vi "Acquisition-Exit.vi"(8 "error in (no error)":errorcluster, 9 "FPGA Ref":T6, 10 "Logging queue element in":T1 {"Ref Dwell time (us)" format="%#.6g"; "Frame Size" items=["100X100"=100, "128X128"=128, "200X200"=200, "256X256"=256, "512X512"=512, "1024x1024"=1024, "2048x2048"=2048]; "Dwell time (us)" format="%#.6g"}, 11 "Logging queue in":T5) -> (0 "error out":errorcluster, 2 "Logging queue element":T1={"Imaging Protocol"=enum."Live Imaging", "Number of Trials"=0, "Frame Size"=512, "# Averaged frames"=0, "Dwell time (us)"=0.0, "Index of Z-plane"=0, "Timelapse?"=FALSE, "Logging process is active"=FALSE, "Speed logging enabled"=FALSE, "tdms file ref"=refnum, "path"=path "", "Trial Number"=0, "Expected # points acquired"=FALSE, "Manually stopped"=FALSE, "Last trial"=FALSE, "Ch0 data"=[], "Ch1 data"=[], "Ref Data"=[], "Ref Frame Time"=[], "Image Time"=[], "Continuous Time"=[], "Ref X Length"=0, "Ref Y Length"=0, "# Ref Averaged frames"=0, "Ref Dwell time (us)"=0.0, "Points acquired"={"Ch0 last trial"=0, "Ch1 last trial"=0, "All trials"=0}, "HW Timings File"=refnum} {"Ref Dwell time (us)" format="%#.6g"; "Frame Size" items=["100X100"=100, "128X128"=128, "200X200"=200, "256X256"=256, "512X512"=512, "1024x1024"=1024, "2048x2048"=2048]; "Dwell time (us)" format="%#.6g"}, 3 "Logging queue out":T5)   [LabVIEW 2017]
doc: "Executes the required code on acquisition exit.\nThis may be at the end of live imaging or at the end of each functional acquisition trial."
uses:
  RIG-SPECIFIC FILES/FPGA Refs/FPGA Ref.ctl
  Typedefs/Logging queue element.ctl
  Typedefs/Imaging Protocols enum.ctl
  Typedefs/Frame Size.ctl
  Typedefs/Acquired points count.ctl
  Typedefs/Data queue ref.ctl
panel:
  in  "Debugging delay":u32
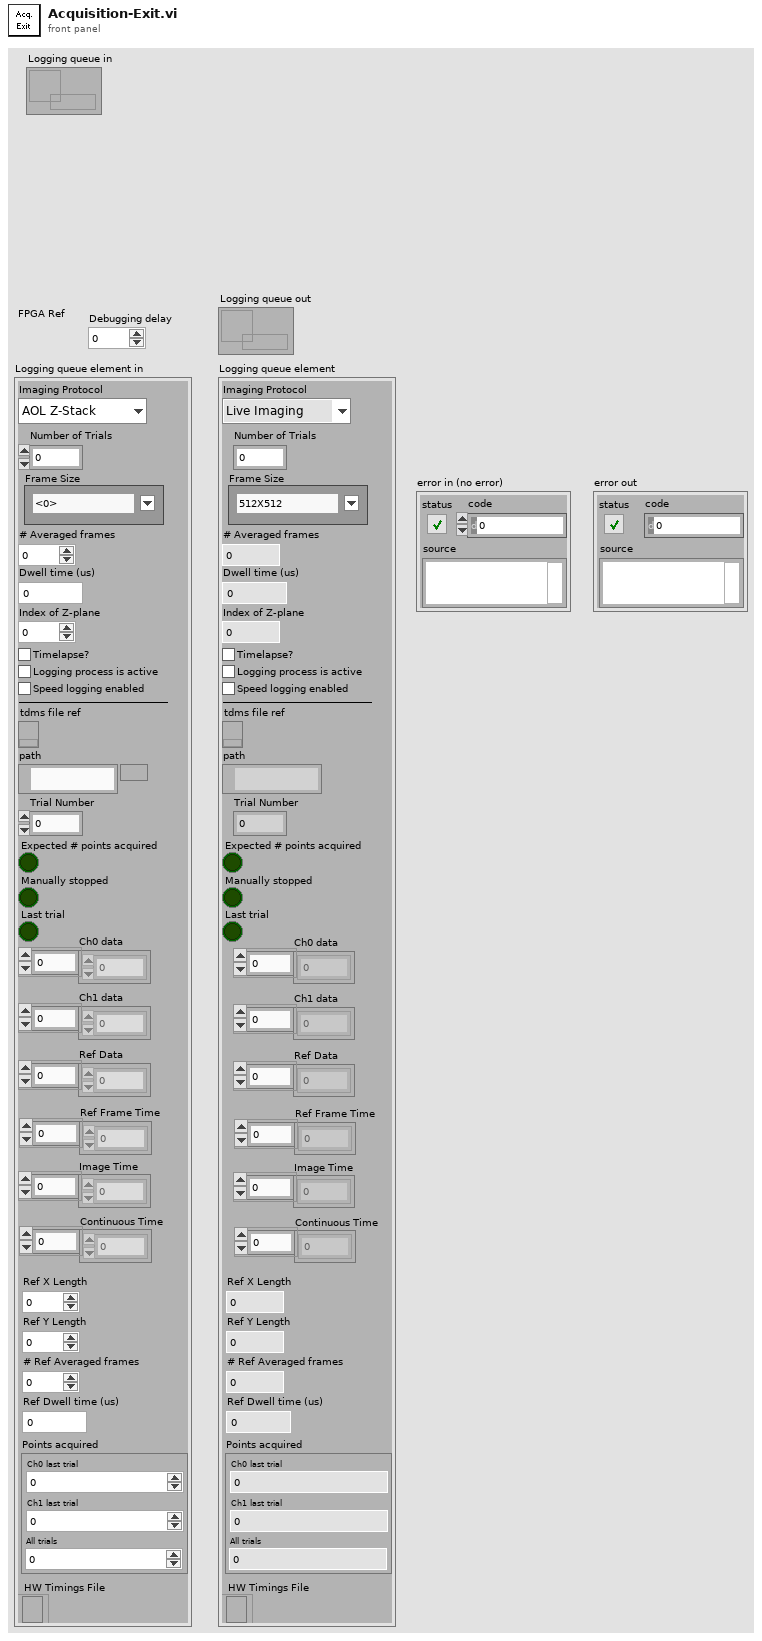
[diagram p1: front panel]
types:
  T1 = typedef "Logging queue element.ctl" = cluster{"Imaging Protocol":T2, "Number of Trials":u16, "Frame Size":T3, "# Averaged frames":u16, "Dwell time (us)":dbl, "Index of Z-plane":i32, "Timelapse?":bool, "Logging process is active":bool, "Speed logging enabled":bool, "tdms file ref":refnum<k34>, "path":path, "Trial Number":i32, "Expected # points acquired":bool, "Manually stopped":bool, "Last trial":bool, "Ch0 data":u32[], "Ch1 data":u32[], "Ref Data":u32[], "Ref Frame Time":u64[], "Image Time":u64[], "Continuous Time":u64[], "Ref X Length":u16, "Ref Y Length":u16, "# Ref Averaged frames":u16, "Ref Dwell time (us)":dbl, "Points acquired":T4, "HW Timings File":refnum<file>}
  T2 = typedef "Imaging Protocols enum.ctl" = enum16{"AOL Z-Stack", "Motor Z Stack", "Functional Acquisition", "Single Plane Acquisition", "Volume Acquisition", "Live Imaging", "Live Plane Imaging", "Live Volume Imaging"}
  T3 = typedef "Frame Size.ctl" = u16
  T4 = typedef "Acquired points count.ctl" = cluster{"Ch0 last trial":u64, "Ch1 last trial":u64, "All trials":u64}
  T5 = typedef "Data queue ref.ctl" = refnum<queue>
  T6 = typedef "FPGA Ref.ctl" = refnum<k20>
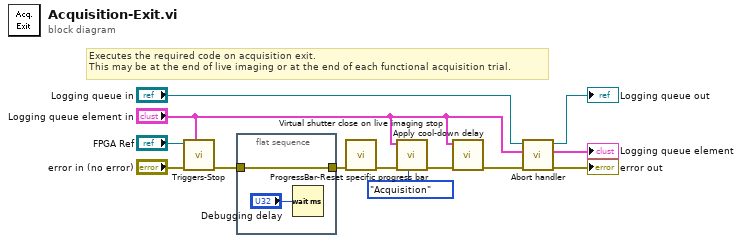
[diagram p0: block diagram]
diagram:
  # "Executes the required code on acquisition exit.\nThis may be at the end of live imaging or at the end of each functional acquisition trial."
  n1 = call "Triggers-Stop.vi"("Logging queue element"="Logging queue element in", "error in (no error)"="error in (no error)", "FPGA Ref"="FPGA Ref") -> ("error out"=w11:errorcluster)  [unwired: 8 in]
  n2 = flat-sequence {
    tunnel: w11 -> [w15]
    tunnel: [w15] -> w12
    frame #0 {
      n3 = Wait (ms)(milliseconds to wait="Debugging delay") -> ()  [unwired: 1 out]
    }
  }
  n4 = call "Virtual shutter close on live imaging stop.vi"("error in (no error)"=w12) -> ("error out"=w10:errorcluster)  [unwired: 10 in]
  n5 = call "ProgressBar-Reset specific progress bar.vi"("Error in"=w10, "Sender"=enum16{"Acquisition", "Logging", "File gen"}."Acquisition", "Z-stack queue cluster"="Logging queue element in") -> ("error out"=w7:errorcluster)  [unwired: 8 in]
  n6 = call "Apply cool-down delay.vi"("error in (no error)"=w7, "Logging queue element in"="Logging queue element in") -> ("error out"=w2:errorcluster)  [unwired: 9 in]
  n7 = call "Abort handler.vi"("error in (no error)"=w2, "Logging queue element in"="Logging queue element in", "Logging queue in"="Logging queue in") -> ("error out"=→"error out":errorcluster, "Logging queue metadata shift out"=→"Logging queue element":T1, "Logging queue out"=→"Logging queue out":T5)  [unwired: 6 in]
